vi "Format pair as connectionList.vi"(10 "channel in":string, 11 "channel 1":string) -> (3 "connectionList":string)   [LabVIEW 2016]
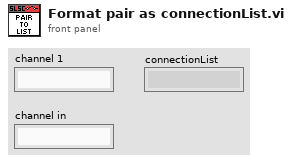
[diagram p1: front panel]
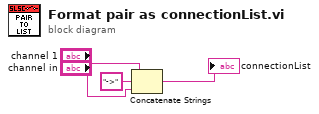
[diagram p0: block diagram]
diagram:
  n1 = Concatenate Strings("channel 1", "->" ("string"), "channel in") -> (→"connectionList":string)
